vi "PCO_GetLookupTableInfo.vi"(0 "ph":u64, 5 "wLUTNum":u16, 11 "error in (no error)":errorcluster {"code" format="%x"}) -> (2 "bOutputWidth":u8, 3 "wIdentifier":u16, 4 "ph out":u64, 6 "ErrorMessage":i32 format="%x", 8 "wNumberOfLuts":u16, 10 "Description":string, 13 "wFormat":u16, 14 "bInputWidth":u8, 15 "error out":errorcluster {"code" format="%x"})   [LabVIEW 2020, in "SDK.lvlib" / "ImageSensor.lvlib"]
doc: "<b>Description:</b>\nDescription of internal lookup tables (LUT) is queried. At first the number of available LUTs in the camera must be queried. This can be done by setting all pointers to NULL despite the pointer to wNumberOffLuts. The value returned in wNumberOffLuts correspondends to the number of available LUTs. Description of a certain LUT can then be queried by calling the function using input parameter wLUTNum and provide valid pointers for the other parameters.\nThe command will be rejected, if Recording State is [run], see PCO_GetRecordingState.\n\n<b>Supported camera type:</b>\npco.edge\n\n<b>Descriptor dependency:</b>\nNone"
uses:
  ImageSensor.lvlib
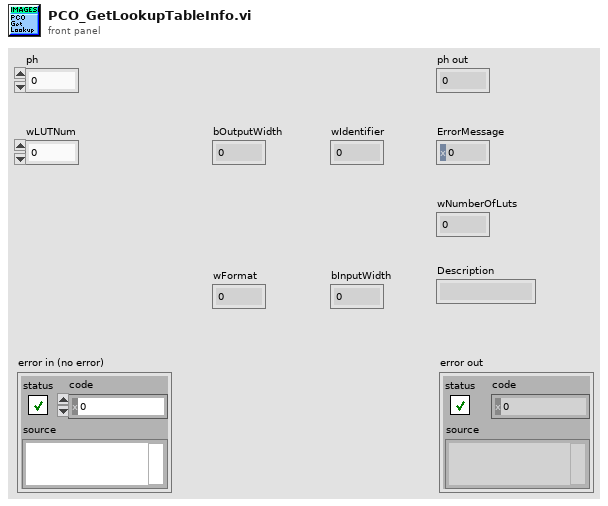
[diagram p1: front panel]
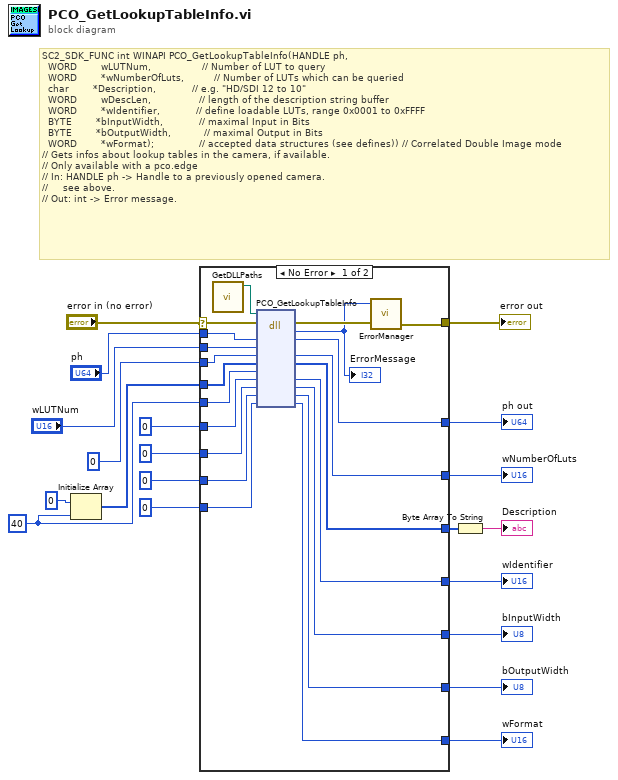
[diagram p0: block diagram]
diagram:
  w14 = u16 40 ("wDescLen")
  # "SC2_SDK_FUNC int WINAPI PCO_GetLookupTableInfo(HANDLE ph,\n  WORD        wLUTNum,                 // Number of LUT to query\n  WORD        *wNumberOfLuts,          // Number of LUTs which can be queried\n  char        *Description,            // e.g. \"HD/SDI 12 to 10\"\n  WORD        wDescLen,                // length of the description string buffer\n  WORD        *wIdentifier,            // define loadable LUTs, range 0x0001 to 0xFFFF\n  BYTE        *bInputWidth,            // maximal Input in Bits\n  BYTE        *bOutputWidth,           // maximal Output in Bits\n  WORD        *wFormat);               // accepted data structures (see defines)) // Correlated Double Image mode\n// Gets infos about lookup tables in the camera, if available.\n// Only available with a pco.edge\n// In: HANDLE ph -> Handle to a previously opened camera.\n//     see above.\n// Out: int -> Error message."
  n1 = Initialize Array(u8 0 ("element"), w14) -> (w15:u8[])
  n2 = case shown="No Error" "error in (no error)" {
    selector: "error in (no error)" -> [w23 w42]
    tunnel: "ph" -> [w41 w49]
    tunnel: [w40 w49] -> w19
    tunnel: "wLUTNum" -> [w39 w48]
    tunnel: u16 0 ("wNumberOfLuts") -> [w22 _]
    tunnel: [w38 w48] -> w16
    tunnel: w15 -> [w37 w47]
    tunnel: w14 -> [w36 _]
    tunnel: [w35 w47] -> w2
    tunnel: u16 0 ("wIdentifier") -> [w34 w46]
    tunnel: [w33 w46] -> w11
    tunnel: u8 0 ("bInputWidth") -> [w32 w45]
    tunnel: [w31 w45] -> w9
    tunnel: u8 0 ("bOutputWidth") -> [w30 w44]
    tunnel: [w29 w44] -> w7
    tunnel: u16 0 ("wFormat") -> [w28 w43]
    tunnel: [w27 w43] -> w5
    tunnel: [w25 w42] -> w4
    frame No Error {
      n3 = call "GetDLLPaths.vi"() -> ("SC2_Cam_Path"=w21:path)  [unwired: 9 in, 2 out]
      n4 = dll-call lib="?" fn="PCO_GetLookupTableInfo"(path in=w21, error in=w23, "ph"=w41, "wLUTNum"=w39, "wNumberOfLuts"=w22, "Description"=w37, "wDescLen"=w36, "wIdentifier"=w34, "bInputWidth"=w32, "bOutputWidth"=w30, "wFormat"=w28) -> (error out=w26:errorcluster, "return type"=w24:i32, "ph"=w40:u64, "wNumberOfLuts"=w38:u16, "Description"=w35:u8[], "wIdentifier"=w33:u16, "bInputWidth"=w31:u8, "bOutputWidth"=w29:u8, "wFormat"=w27:u16)  [unwired: 3 in, 1 out]
      "ErrorMessage" <- w24
      n5 = call "ErrorManager.vi"("error in (no error)"=w26, "error code"=w24) -> ("error out"=w25:errorcluster)  [unwired: 3 in]
    }
    frame Error {
    }
  }
  "ph out" <- w19
  "wNumberOfLuts" <- w16
  "wIdentifier" <- w11
  "bInputWidth" <- w9
  "bOutputWidth" <- w7
  "wFormat" <- w5
  "error out" <- w4
  n6 = Byte Array To String(unsigned byte array=w2) -> (string=→"Description":string)
